vi "getParameters.vi"(11 "EnterMaintenanceCommand in":refnum<class "EnterMaintenanceCommand.lvclass">) -> (2 "Parameters":T1, 3 "EnterMaintenanceCommand out":refnum<class "EnterMaintenanceCommand.lvclass">)   [LabVIEW 2016, in "EnterMaintenanceCommand.lvclass"]
uses:
  EnterMaintenanceCommand.lvclass
  DataTypes/Topics/CommandEnterMaintenance.ctl
  DataTypes/Topics/Parts/CommandId.ctl
  EnterMaintenanceCommand.lvclass/EnterMaintenanceCommand.ctl
  DataTypes/Topics/M1M3SupportTopics.lvlib
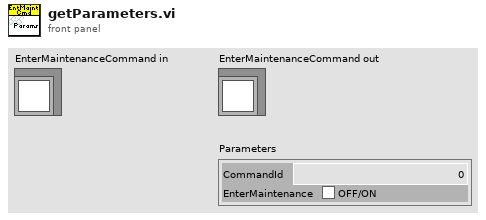
[diagram p1: front panel]
types:
  T1 = typedef "M1M3SupportTopics.lvlib/CommandEnterMaintenance.ctl" = cluster{"CommandId":T2, "EnterMaintenance":bool}
  T2 = typedef "M1M3SupportTopics.lvlib/CommandId.ctl" = i32
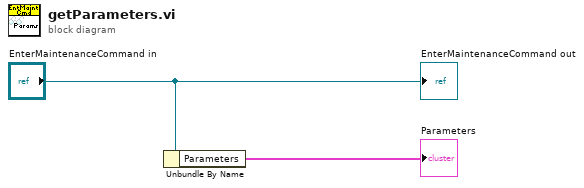
[diagram p0: block diagram]
diagram:
  n1 = Unbundle By Name("EnterMaintenanceCommand in") -> ("Parameters"=→"Parameters":T1)
  "EnterMaintenanceCommand out" <- "EnterMaintenanceCommand in"
